vi "DMAGenerator.vi"(4 "Counter_TimerOutputs":T6, 5 "DutyCycleOutputs":T5, 6 "Encoder_TimerOutputs":T1, 7 "Counter_Outputs":T7, 8 "Encoder_Outputs":T3, 9 "DigitalInputs":u32, 10 "AnalogInputs":u16[](array[numeric])=[0, 0, 0, 0, 0, 0, 0, 0], 11 "AnalogTriggerOutputs":T9) -> (2 "NewDataLength":u8, 3 "NewData":u32[](array[numeric]))   [LabVIEW 2019]
uses:
  Controls/AnalogTrigger_Outputs.ctl
  Helpers/AnalogTriggerOutput.ctl
  Controls/Counter_Outputs.ctl
  Controls/Counter_Output.ctl
  Controls/Counter_TimerOutputs.ctl
  Helpers/TimerOutput.ctl
  Controls/DutyCycle_Outputs.ctl
  Controls/Encoder_Outputs.ctl
  Controls/Encoder_Output.ctl
  Controls/Encoder_TimerOutputs.ctl
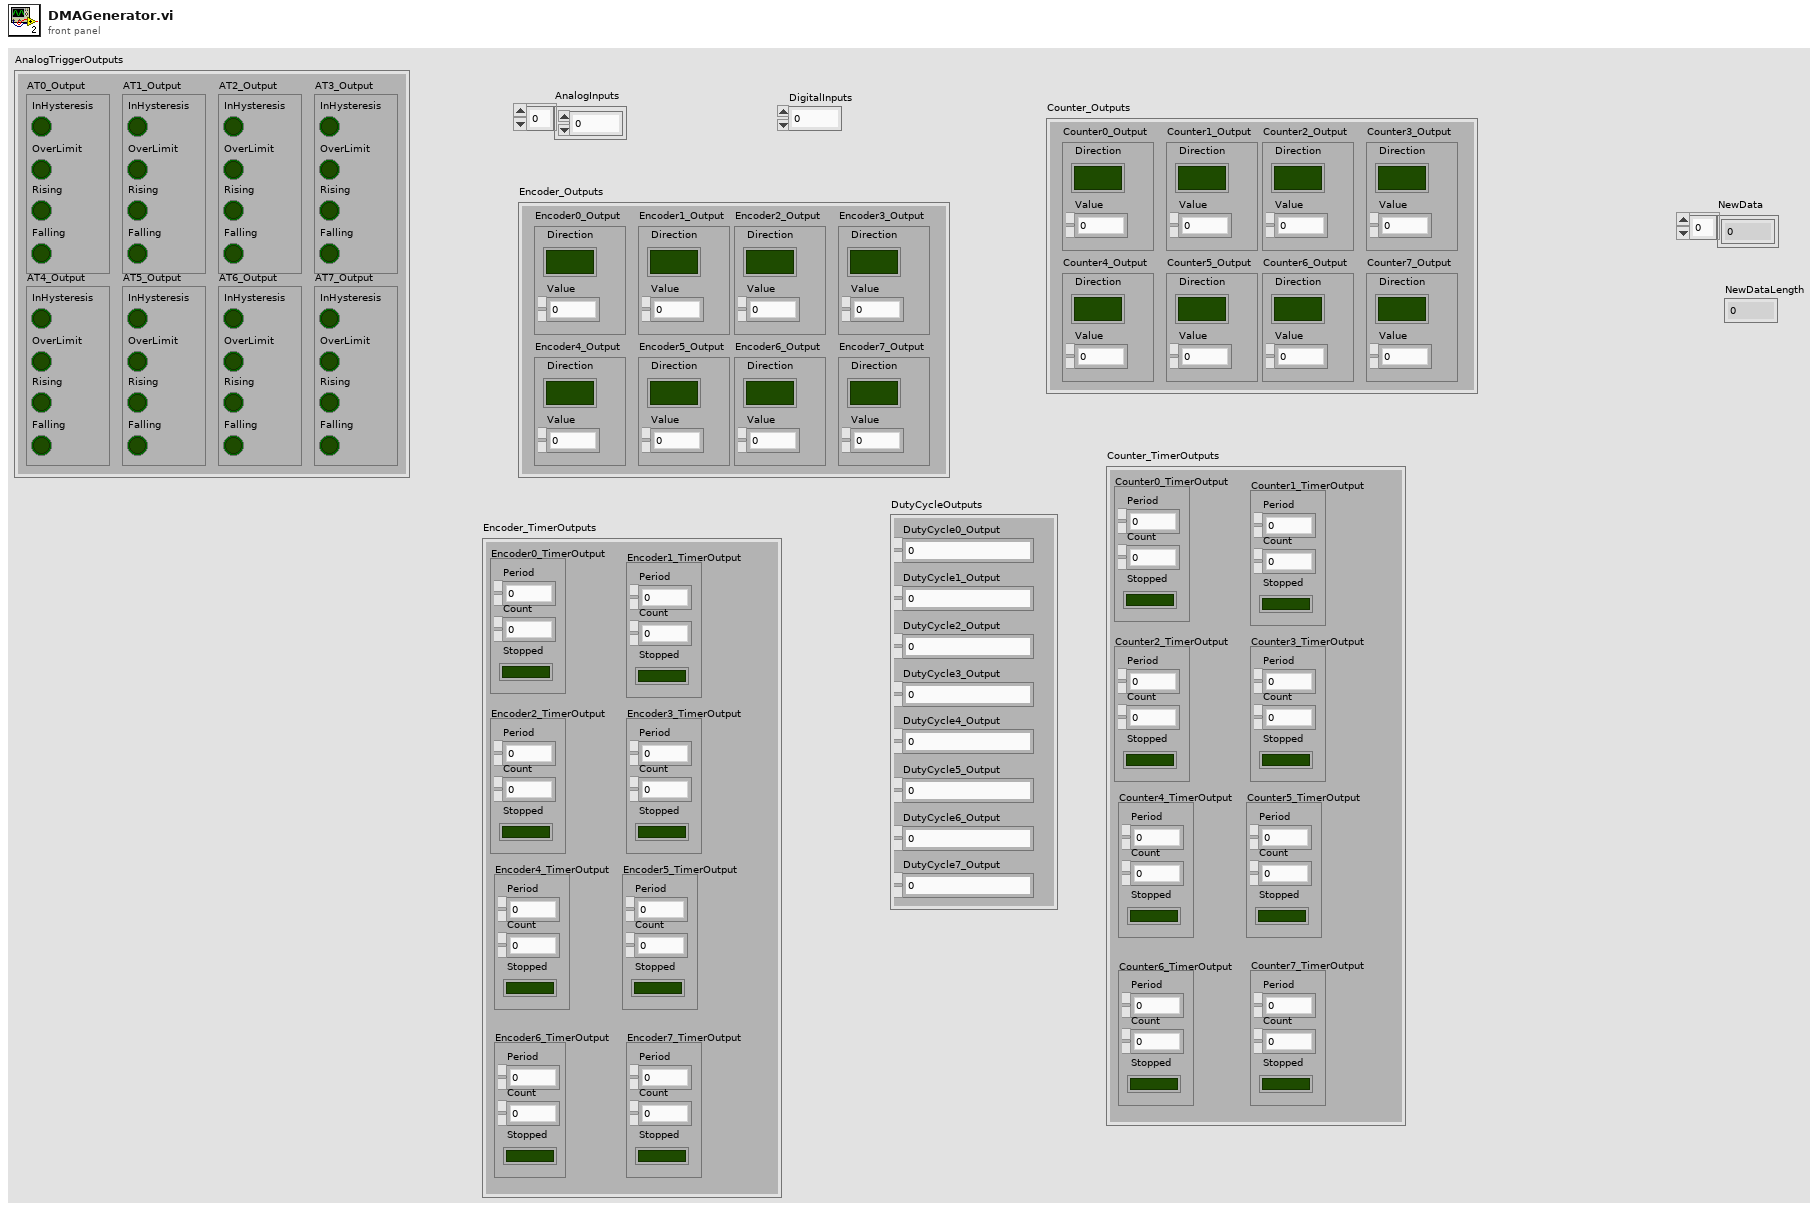
[diagram p1: front panel]
types:
  T1 = typedef "Encoder_TimerOutputs.ctl" = cluster{"Encoder0_TimerOutput":T2, "Encoder1_TimerOutput":T2, "Encoder2_TimerOutput":T2, "Encoder3_TimerOutput":T2, "Encoder4_TimerOutput":T2, "Encoder5_TimerOutput":T2, "Encoder6_TimerOutput":T2, "Encoder7_TimerOutput":T2}
  T2 = typedef "TimerOutput.ctl" = cluster{"Period":fxp<+,24,25>, "Count":i16, "Stopped":bool}
  T3 = typedef "Encoder_Outputs.ctl" = cluster{"Encoder0_Output":T4, "Encoder1_Output":T4, "Encoder2_Output":T4, "Encoder3_Output":T4, "Encoder4_Output":T4, "Encoder5_Output":T4, "Encoder6_Output":T4, "Encoder7_Output":T4}
  T4 = typedef "Encoder_Output.ctl" = cluster{"Direction":bool, "Value":fxp<+/-,31,31>}
  T5 = typedef "DutyCycle_Outputs.ctl" = cluster{"DutyCycle0_Output":fxp<+,31,31>, "DutyCycle1_Output":fxp<+,31,31>, "DutyCycle2_Output":fxp<+,31,31>, "DutyCycle3_Output":fxp<+,31,31>, "DutyCycle4_Output":fxp<+,31,31>, "DutyCycle5_Output":fxp<+,31,31>, "DutyCycle6_Output":fxp<+,31,31>, "DutyCycle7_Output":fxp<+,31,31>}
  T6 = typedef "Counter_TimerOutputs.ctl" = cluster{"Counter0_TimerOutput":T2, "Counter1_TimerOutput":T2, "Counter2_TimerOutput":T2, "Counter3_TimerOutput":T2, "Counter4_TimerOutput":T2, "Counter5_TimerOutput":T2, "Counter6_TimerOutput":T2, "Counter7_TimerOutput":T2}
  T7 = typedef "Counter_Outputs.ctl" = cluster{"Counter0_Output":T8, "Counter1_Output":T8, "Counter2_Output":T8, "Counter3_Output":T8, "Counter4_Output":T8, "Counter5_Output":T8, "Counter6_Output":T8, "Counter7_Output":T8}
  T8 = typedef "Counter_Output.ctl" = cluster{"Direction":bool, "Value":fxp<+/-,31,31>}
  T9 = typedef "AnalogTrigger_Outputs.ctl" = cluster{"AT0_Output":T10, "AT1_Output":T10, "AT2_Output":T10, "AT3_Output":T10, "AT4_Output":T10, "AT5_Output":T10, "AT6_Output":T10, "AT7_Output":T10}
  T10 = typedef "AnalogTriggerOutput.ctl" = cluster{"InHysteresis":bool, "OverLimit":bool, "Rising":bool, "Falling":bool}
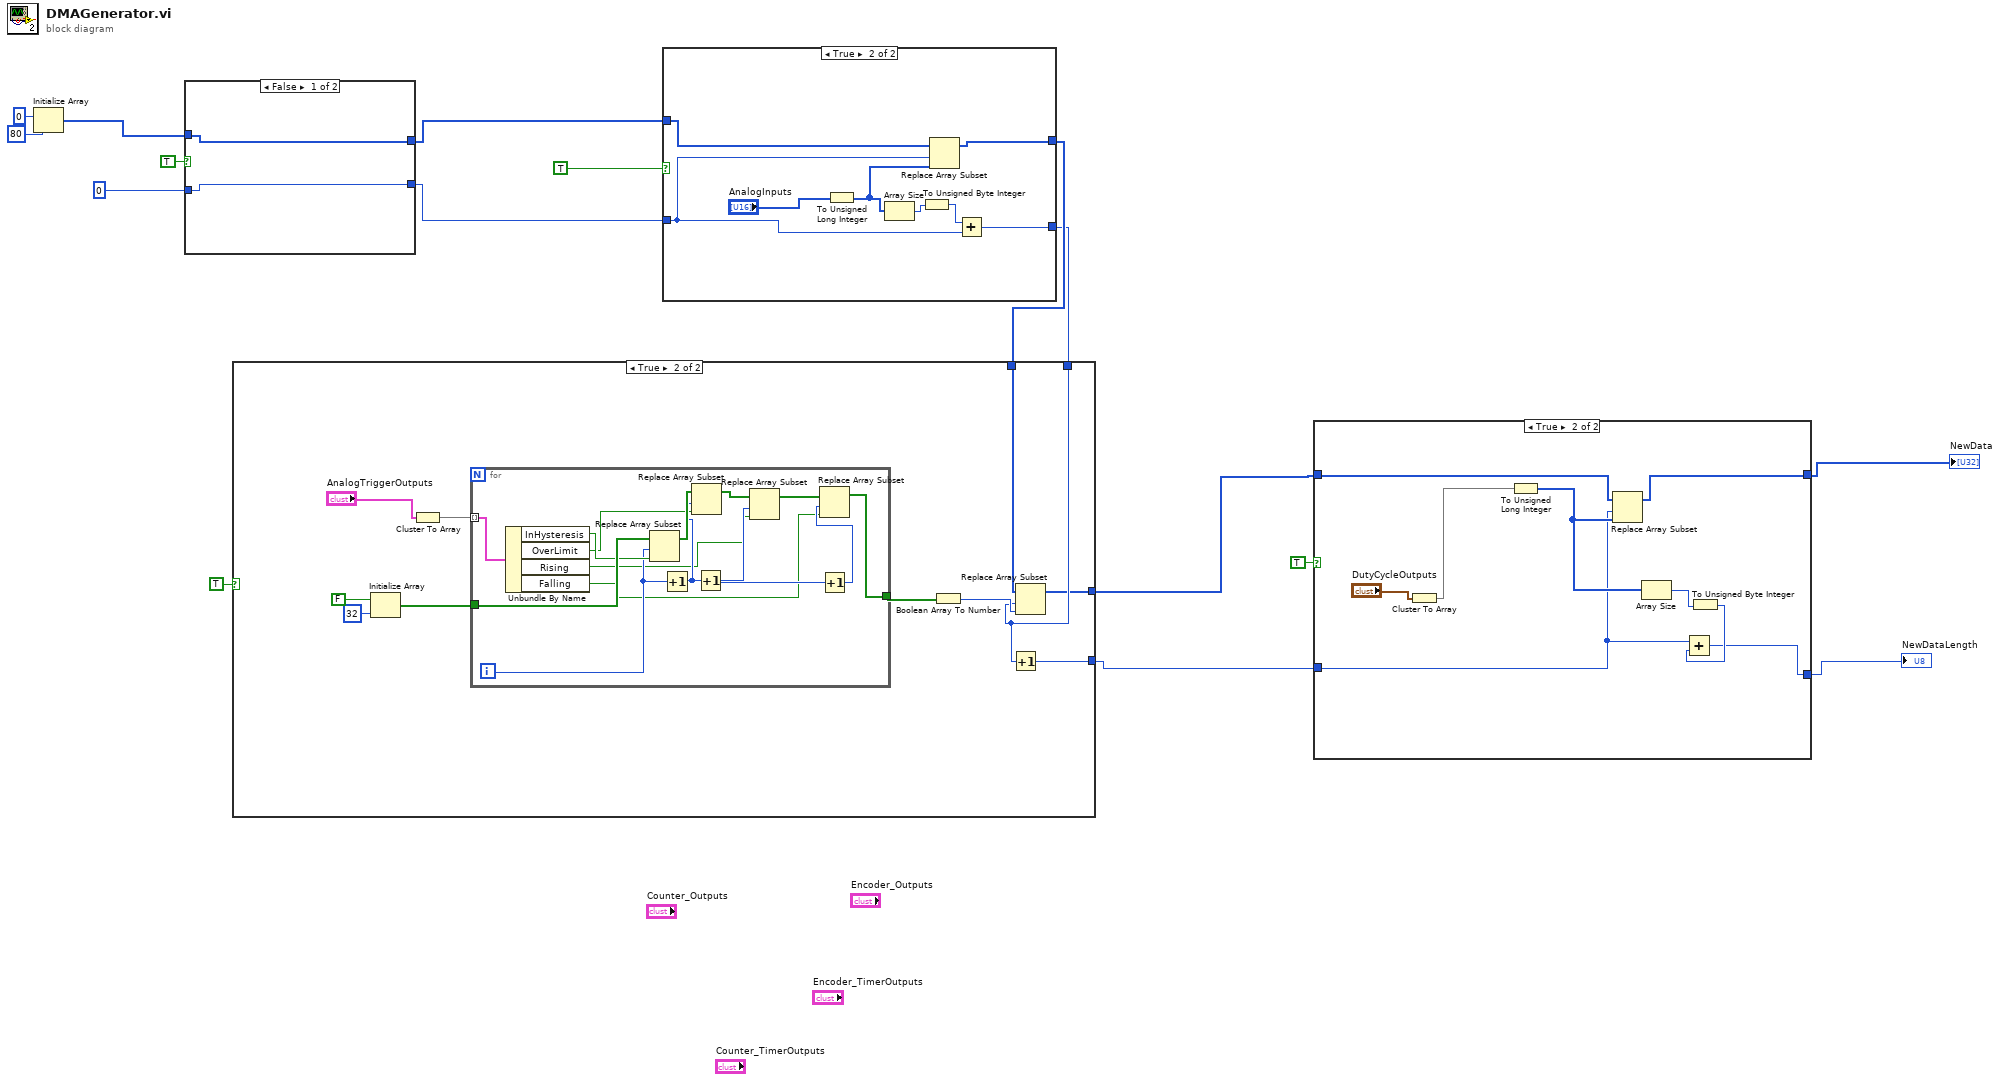
[diagram p0: block diagram]
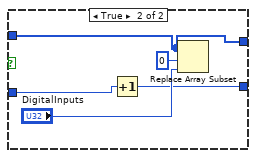
[diagram p5: hidden frame]
diagram:
  n1 = Initialize Array(u32 0 ("element"), 80 ("dimension size")) -> (w14:u32[])
  n2 = case shown="False" TRUE {
    tunnel: w14 -> [w18 w21]
    tunnel: [w18 w21] -> w9
    tunnel: u8 0 -> [w17 w20]
    tunnel: [w17 w19] -> w10
    frame False {
    }
    frame True {
      n3 = Increment(x=w20) -> (x+1=w19:u8)
      n4 = Replace Array Subset(array=w21, new element="DigitalInputs", index=0) -> ()  [unwired: 1 out]
    }
  }
  n5 = case shown="True" TRUE {
    tunnel: w10 -> [w24 w30]
    tunnel: w9 -> [w25 w31]
    tunnel: [w24 w29] -> w6
    tunnel: [w25 w28] -> w7
    frame False {
    }
    frame True {
      n6 = To Unsigned Long Integer(number="AnalogInputs") -> (unsigned 32bit integer=w32:u32[])
      n7 = Array Size(array=w32) -> (size(s)=w27:i32)
      n8 = To Unsigned Byte Integer(number=w27) -> (unsigned 8bit integer=w26:u8)
      n9 = Replace Array Subset(array=w31, new element=w32, index=w30) -> (w28:u32[])
      n10 = Add(x=w26, y=w30) -> (x+y=w29:u8)
    }
  }
  n11 = case shown="True" TRUE {
    tunnel: w7 -> [w34 w39]
    tunnel: w6 -> [w35 w38]
    tunnel: [w35 w37] -> w3
    tunnel: [w34 w36] -> w4
    frame False {
    }
    frame True {
      n12 = Initialize Array(FALSE, 32 ("dimension size")) -> (w42:bool[])
      n13 = Cluster To Array(cluster="AnalogTriggerOutputs") -> (array=w45:T10[])
      n14 = for {
        tunnel: w45 -> [w60] mode=indexing
        tunnel: w42 -> [w59]
        tunnel: [w53] -> w41
        i -> [w57]
        n15 = Unbundle By Name(w60) -> ("InHysteresis"=w58:bool, "OverLimit"=w47:bool, "Rising"=w48:bool, "Falling"=w49:bool)
        n16 = Replace Array Subset(array=w59, new element=w58, index=w57) -> (w56:bool[])
        n17 = Increment(x=w57) -> (x+1=w52:i32)
        n18 = Replace Array Subset(array=w56, new element=w47, index=w52) -> (w55:bool[])
        n19 = Increment(x=w52) -> (x+1=w51:i32)
        n20 = Replace Array Subset(array=w55, new element=w48, index=w51) -> (w54:bool[])
        n21 = Increment(x=w51) -> (x+1=w50:i32)
        n22 = Replace Array Subset(array=w54, new element=w49, index=w50) -> (w53:bool[])
      }
      n23 = Boolean Array To Number(Boolean array=w41) -> (number=w40:u32)
      n24 = Increment(x=w38) -> (x+1=w37:u8)
      n25 = Replace Array Subset(array=w39, new element=w40, index=w38) -> (w36:u32[])
    }
  }
  n26 = case shown="True" TRUE {
    tunnel: w4 -> [w62 w69]
    tunnel: w3 -> [w61 w66]
    tunnel: [w62 w63] -> w2
    tunnel: [w61 w64] -> w1
    frame False {
    }
    frame True {
      n27 = Cluster To Array(cluster="DutyCycleOutputs") -> (array=w70:fxp<+,31,31>[])
      n28 = To Unsigned Long Integer(number=w70) -> (unsigned 32bit integer=w68:u32[])
      n29 = Replace Array Subset(array=w69, new element=w68, index=w66) -> (w63:u32[])
      n30 = Array Size(array=w68) -> (size(s)=w67:i32)
      n31 = To Unsigned Byte Integer(number=w67) -> (unsigned 8bit integer=w65:u8)
      n32 = Add(x=w66, y=w65) -> (x+y=w64:u8)
    }
  }
  "NewData" <- w2
  "NewDataLength" <- w1
